vi "get_c_v.vi"(4 "error in":errorcluster, 5 "viShortPath":string, 6 "controlName":string, 7 "ApplicationRef In":refnum<k7>) -> (0 "error out":errorcluster, 2 "ControlValue":variant, 3 "ApplicationRefOut":refnum<k7>)   [LabVIEW 2010]
panel:
  out "concatenated string":string
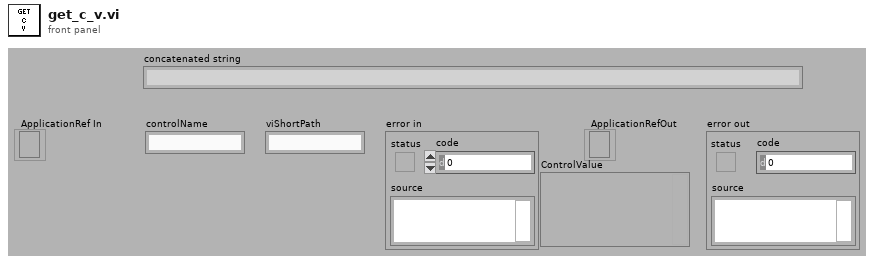
[diagram p1: front panel]
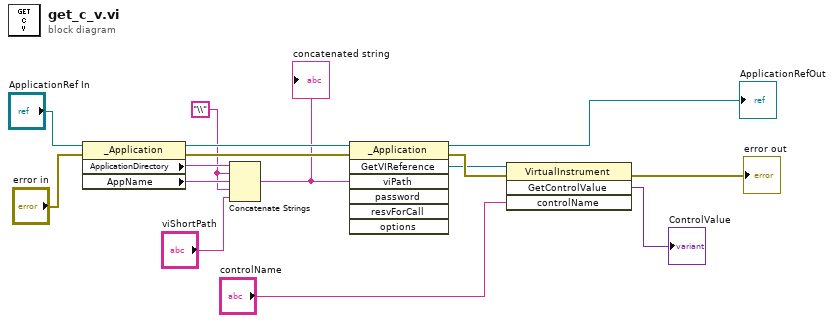
[diagram p0: block diagram]
diagram:
  w4 = "\\"
  n1 = property class="_Application"(reference="ApplicationRef In", error in="error in") -> (reference out=w8:refnum<k7>, error out=w7:errorcluster, "ApplicationDirectory"=w6:string, "AppName"=w5:string)
  n2 = Concatenate Strings(w6, w4, w5, w4, "viShortPath") -> (w1:string)
  "concatenated string" <- w1
  n3 = invoke class="_Application" method="GetVIReference"(reference=w8, error in=w7, "viPath"=w1) -> (reference out=→"ApplicationRefOut":refnum<k7>, error out=w14:errorcluster, "GetVIReference"=w12:refnum<k7>)  [unwired: 4 in, 4 out]
  n4 = invoke class="VirtualInstrument" method="GetControlValue"(reference=w12, error in=w14, "controlName"="controlName") -> (error out=→"error out":errorcluster, "GetControlValue"=→"ControlValue":variant)  [unwired: 1 in, 2 out]
